vi "read data.vi"(8 "error in (no error)":errorcluster, 11 "Processor in":refnum<class "Processor.lvclass">) -> (0 "error out":errorcluster, 2 "data":dbl, 3 "Processor out":refnum<class "Processor.lvclass">)   [LabVIEW 2025, in "Processor.lvclass"]
uses:
  Processor.lvclass
  Processor.lvclass/Processor.ctl
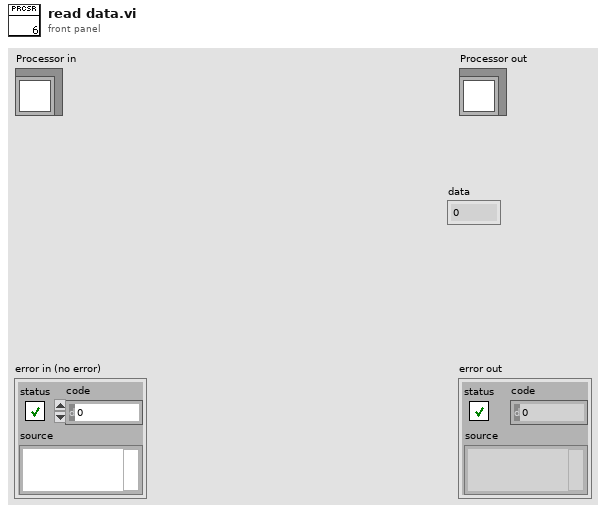
[diagram p1: front panel]
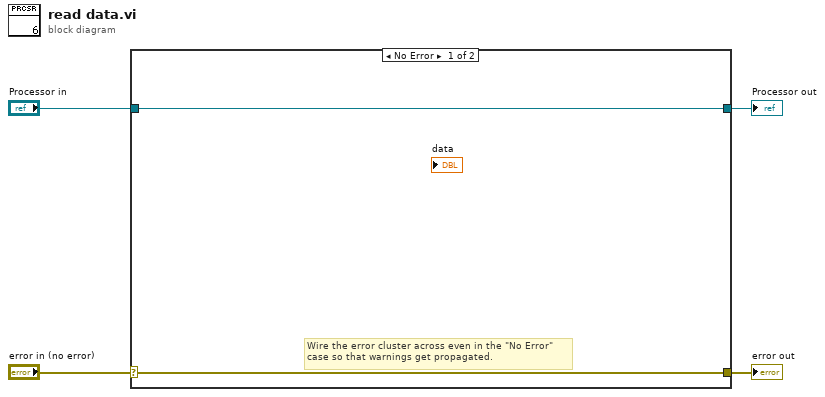
[diagram p0: block diagram]
diagram:
  n1 = case shown="No Error" "error in (no error)" {
    selector: "error in (no error)" -> [w5 w8]
    tunnel: [w5 w8] -> w3
    tunnel: [w6 w7] -> w1
    tunnel: "Processor in" -> [w6 w7]
    frame No Error {
      # "Wire the error cluster across even in the \"No Error\"\ncase so that warnings get propagated."
    }
    frame Error {
    }
  }
  "error out" <- w3
  "Processor out" <- w1
